vi "store2ADCToFileAll2.vi"(0 "ADCselect":enum16{"ADC18", "ADC16", "2ADC", "None"}(ring)=enum."2ADC", 1 "Test type":T1(ring), 2 "attenuateVal":u16, 3 "iterationXtalk":u32, 4 "keithleyVoltage":dbl) -> (5 "outputFileName":string, 6 "error out":errorcluster)   [LabVIEW 2014]
uses:
  Global 1.vi
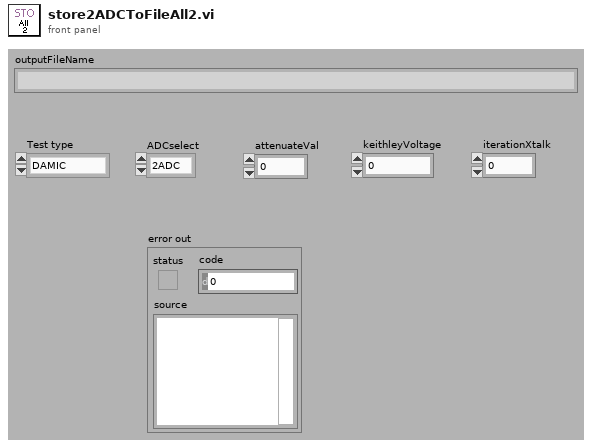
[diagram p1: front panel]
types:
  T1 = enum16{"DAMIC", "NOISE", "GAIN", "LINEAR18", "XTALK", "TEMP", "LINEAR16", "CONSO"}
  T2 = enum16{"open", "replace", "create", "open or create", "replace or create", "replace or create with confirmation"}
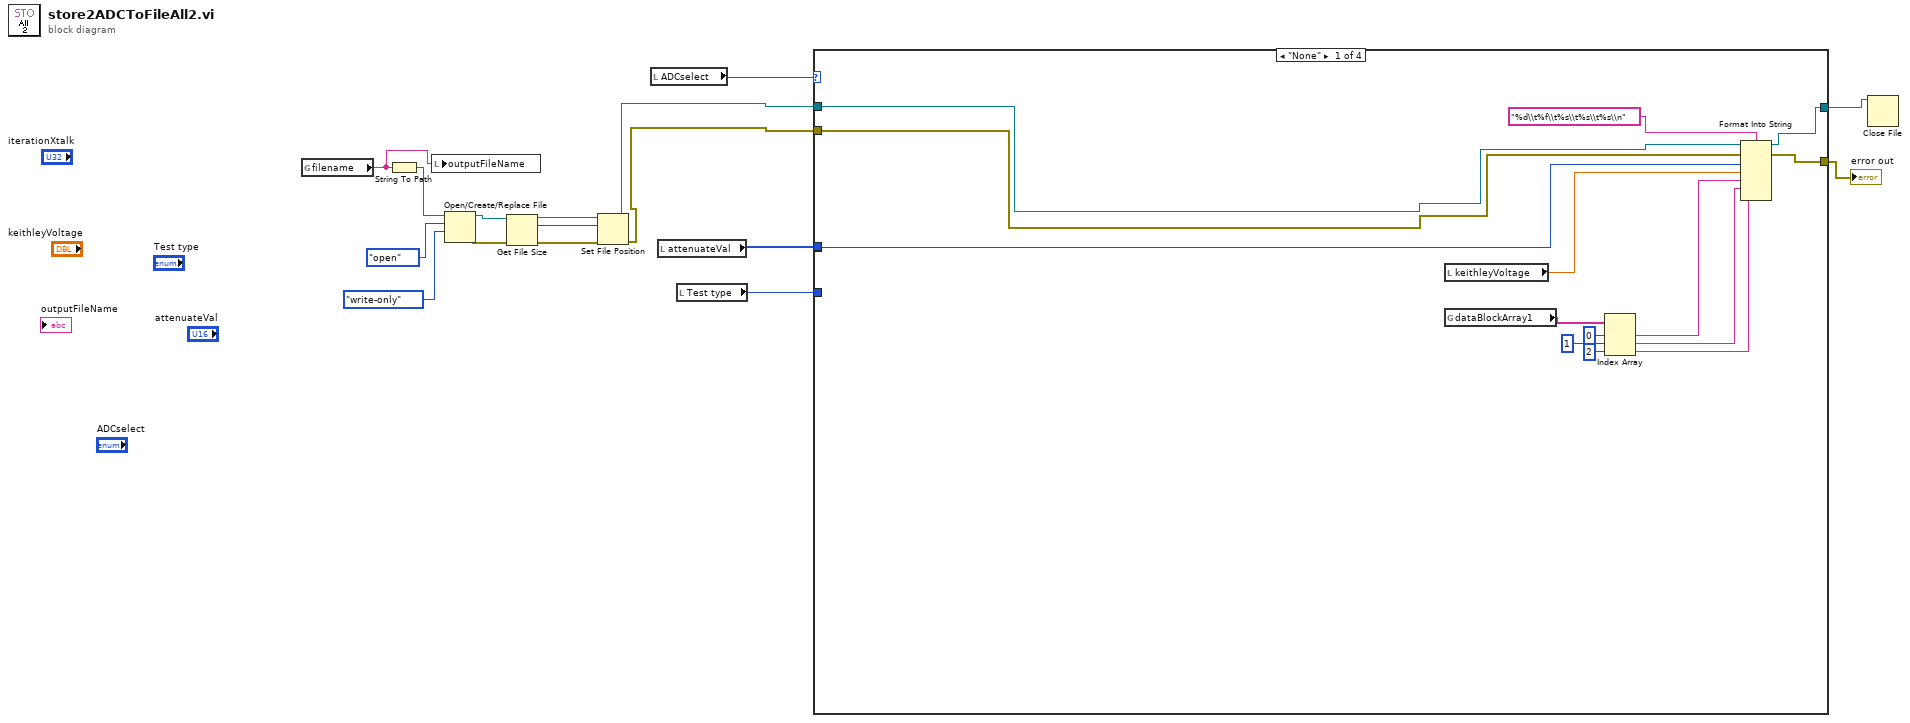
[diagram p0: block diagram]
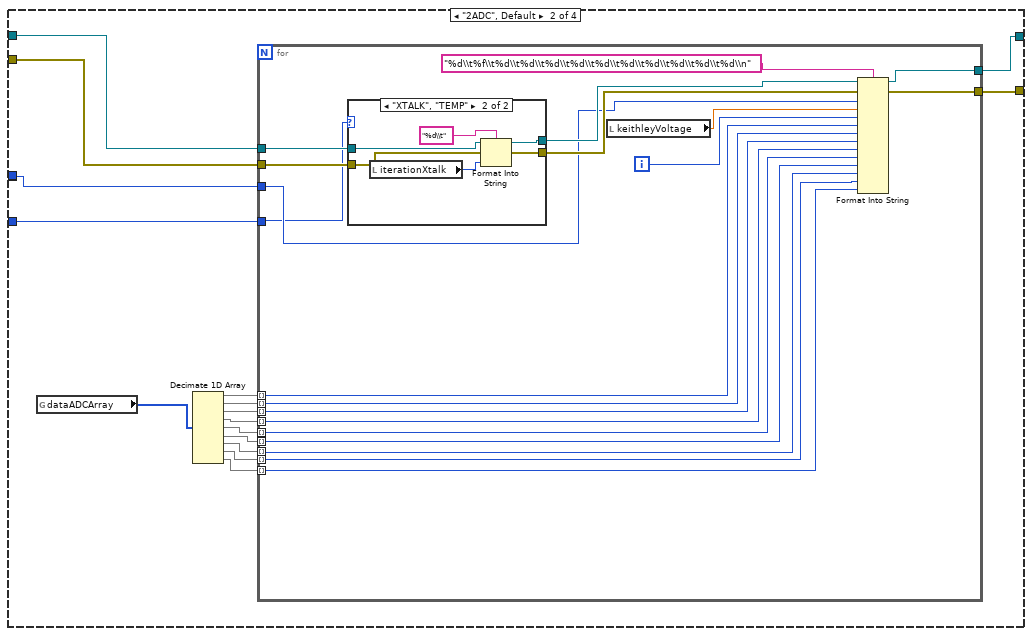
[diagram p2: hidden frame]
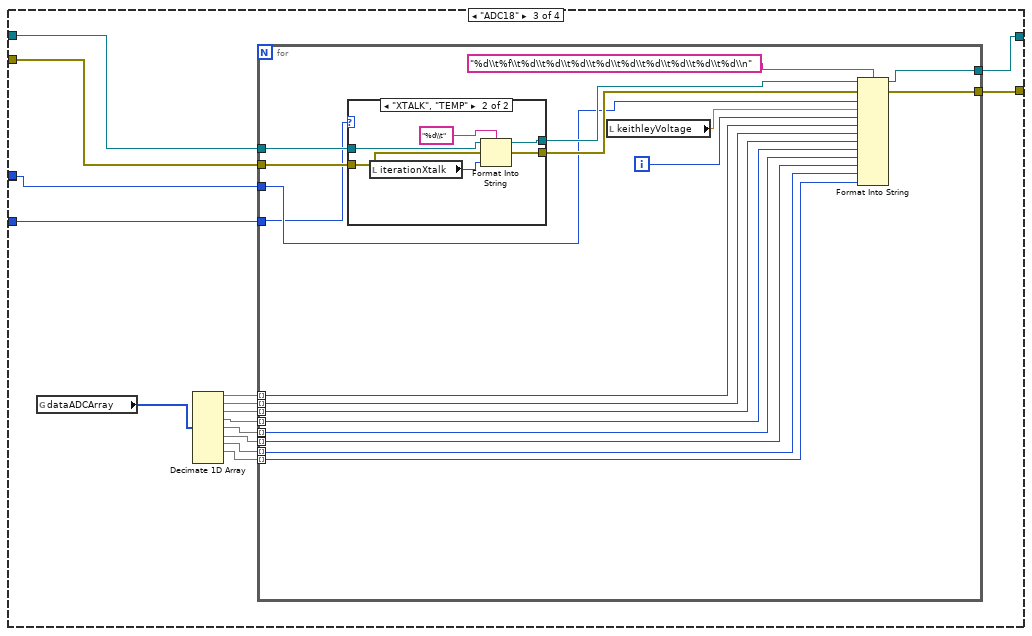
[diagram p4: hidden frame]
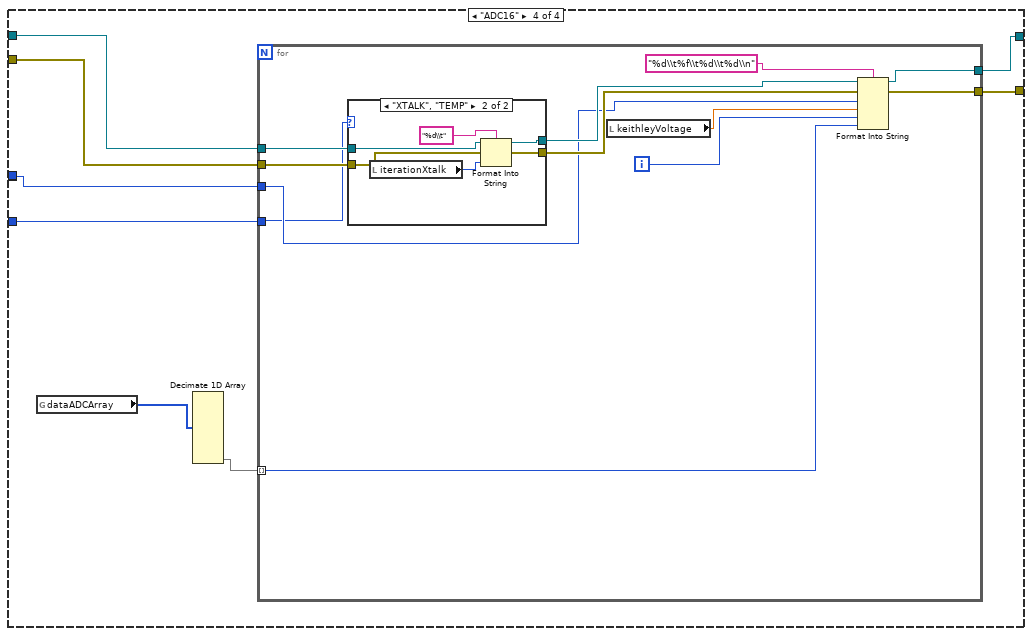
[diagram p6: hidden frame]
diagram:
  n1 = global read "Global 1.vi" "filename"() -> (w14:string)
  n2 = String To Path(string=w14) -> (path=w8:path)
  n3 = local write "outputFileName"(w14) -> ()
  n4 = Open/Create/Replace File(file path (use dialog)=w8, operation (0:open)=T2."open", access (0:read/write)=enum16{"read/write", "read-only", "write-only"}."write-only") -> (refnum out=w10:refnum<file>, error out=w11:errorcluster)  [unwired: 1 in, 3 out]
  n5 = Get File Size(file=w10, error in=w11) -> (refnum out=w13:refnum<file>, size (in bytes)=w6:i64, 0:w12:errorcluster)
  n6 = Set File Position(offset (in bytes) (0)=w6, refnum=w13, error in=w12) -> (refnum out=w16:refnum<file>, error out=w15:errorcluster)  [unwired: 1 out]
  n7 = local read "ADCselect"() -> (w5:enum16{"ADC18", "ADC16", "2ADC", "None"})
  n8 = local read "attenuateVal"() -> (w4:u16)
  n9 = local read "Test type"() -> (w3:T1)
  n10 = case shown="\"None\"" w5 {
    tunnel: w15 -> [w30 w46 w89 w124]
    tunnel: w16 -> [w29 w45 w88 w123]
    tunnel: [w28 w44 w87 w122] -> w2
    tunnel: [w27 w43 w86 w121] -> w1
    tunnel: w4 -> [w26 w42 w85 w120]
    tunnel: w4 -> [_ _ _ _]
    tunnel: w3 -> [_ w41 w84 w119]
    frame "None" {
      n11 = local read "keithleyVoltage"() -> (w24:dbl)
      n12 = global read "Global 1.vi" "dataBlockArray1"() -> (w23:string[])
      n13 = Index Array(array=w23, index #1=0 ("index"), index #2=1 ("index"), index #3=2 ("index")) -> (element #1=w22:string, element #2=w18:string, element #3=w17:string)
      n14 = Format Into String(format string="%d\\t%f\\t%s\\t%s\\t%s\\n", initial string=w29, error in=w30, w26, w24, w22, w18, w17) -> (resulting string=w28:refnum<file>, error out=w27:errorcluster)
    }
    frame "2ADC", Default {
      n15 = global read "Global 1.vi" "dataADCArray"() -> (w40:i32[])
      n16 = Decimate 1D Array(w40) -> (w39:i32[], w38:i32[], w37:i32[], w36:i32[], w35:i32[], w34:i32[], w33:i32[], w32:i32[], w31:i32[])
      n17 = for {
        tunnel: w46 -> [w62]
        tunnel: w45 -> [w63]
        tunnel: [w65] -> w44
        tunnel: [w64] -> w43
        tunnel: w42 -> [w58]
        tunnel: w41 -> [w57]
        tunnel: w39 -> [w55] mode=indexing
        tunnel: w38 -> [w54] mode=indexing
        tunnel: w37 -> [w53] mode=indexing
        tunnel: w36 -> [w52] mode=indexing
        tunnel: w35 -> [w51] mode=indexing
        tunnel: w34 -> [w50] mode=indexing
        tunnel: w33 -> [w49] mode=indexing
        tunnel: w32 -> [w48] mode=indexing
        tunnel: w31 -> [w47] mode=indexing
        i -> [w56]
        n18 = case shown="\"XTALK\", \"TEMP\"" w57 {
          tunnel: w63 -> [w68 w74]
          tunnel: w62 -> [w67 w73]
          tunnel: [w68 w72] -> w61
          tunnel: [w67 w71] -> w60
          frame "NOISE", Default {
          }
          frame "XTALK", "TEMP" {
            n19 = local read "iterationXtalk"() -> (w69:u32)
            n20 = Format Into String(format string="%d\\t", initial string=w74, error in=w73, w69) -> (resulting string=w72:refnum<file>, error out=w71:errorcluster)
          }
        }
        n21 = local read "keithleyVoltage"() -> (w59:dbl)
        n22 = Format Into String(format string="%d\\t%f\\t%d\\t%d\\t%d\\t%d\\t%d\\t%d\\t%d\\t%d\\t%d\\t%d\\n", initial string=w61, error in=w60, w58, w59, w56, w55, w54, w53, w52, w51, w50, w49, w48, w47) -> (resulting string=w65:refnum<file>, error out=w64:errorcluster)
      }
    }
    frame "ADC18" {
      n23 = global read "Global 1.vi" "dataADCArray"() -> (w83:i32[])
      n24 = Decimate 1D Array(w83) -> (w82:i32[], w81:i32[], w80:i32[], w79:i32[], w78:i32[], w77:i32[], w76:i32[], w75:i32[])  [unwired: 1 out]
      n25 = for {
        tunnel: w89 -> [w104]
        tunnel: w88 -> [w105]
        tunnel: [w107] -> w87
        tunnel: [w106] -> w86
        tunnel: w85 -> [w100]
        tunnel: w84 -> [w99]
        tunnel: w82 -> [w97] mode=indexing
        tunnel: w81 -> [w96] mode=indexing
        tunnel: w80 -> [w95] mode=indexing
        tunnel: w79 -> [w94] mode=indexing
        tunnel: w78 -> [w93] mode=indexing
        tunnel: w77 -> [w92] mode=indexing
        tunnel: w76 -> [w91] mode=indexing
        tunnel: w75 -> [w90] mode=indexing
        i -> [w98]
        n26 = case shown="\"XTALK\", \"TEMP\"" w99 {
          tunnel: w105 -> [w110 w116]
          tunnel: w104 -> [w109 w115]
          tunnel: [w110 w114] -> w103
          tunnel: [w109 w113] -> w102
          frame "NOISE", Default {
          }
          frame "XTALK", "TEMP" {
            n27 = local read "iterationXtalk"() -> (w111:u32)
            n28 = Format Into String(format string="%d\\t", initial string=w116, error in=w115, w111) -> (resulting string=w114:refnum<file>, error out=w113:errorcluster)
          }
        }
        n29 = local read "keithleyVoltage"() -> (w101:dbl)
        n30 = Format Into String(format string="%d\\t%f\\t%d\\t%d\\t%d\\t%d\\t%d\\t%d\\t%d\\t%d\\t%d\\n", initial string=w103, error in=w102, w100, w101, w98, w97, w96, w95, w94, w93, w92, w91, w90) -> (resulting string=w107:refnum<file>, error out=w106:errorcluster)
      }
    }
    frame "ADC16" {
      n31 = global read "Global 1.vi" "dataADCArray"() -> (w118:i32[])
      n32 = Decimate 1D Array(w118) -> (w117:i32[])  [unwired: 8 out]
      n33 = for {
        tunnel: w124 -> [w132]
        tunnel: w123 -> [w133]
        tunnel: [w135] -> w122
        tunnel: [w134] -> w121
        tunnel: w120 -> [w128]
        tunnel: w119 -> [w127]
        tunnel: w117 -> [w125] mode=indexing
        i -> [w126]
        n34 = case shown="\"XTALK\", \"TEMP\"" w127 {
          tunnel: w133 -> [w138 w144]
          tunnel: w132 -> [w137 w143]
          tunnel: [w138 w142] -> w131
          tunnel: [w137 w141] -> w130
          frame "NOISE", Default {
          }
          frame "XTALK", "TEMP" {
            n35 = local read "iterationXtalk"() -> (w139:u32)
            n36 = Format Into String(format string="%d\\t", initial string=w144, error in=w143, w139) -> (resulting string=w142:refnum<file>, error out=w141:errorcluster)
          }
        }
        n37 = local read "keithleyVoltage"() -> (w129:dbl)
        n38 = Format Into String(format string="%d\\t%f\\t%d\\t%d\\n", initial string=w131, error in=w130, w128, w129, w126, w125) -> (resulting string=w135:refnum<file>, error out=w134:errorcluster)
      }
    }
  }
  "error out" <- w1
  n39 = Close File(refnum=w2) -> ()  [unwired: 1 in, 2 out]
